vi "Do Turn.vi"(6 "Team in":refnum<class "Team.lvclass">, 7 "Round Number":u32, 9 "Neighbors":i32[](array[numeric]), 10 "Position":T1, 11 "Square in":refnum<class "Square.lvclass">) -> (2 "Run Result":T2, 3 "Square out":refnum<class "Square.lvclass">, 4 "Team out":refnum<class "Team.lvclass">)   [LabVIEW 2020, in "SquareBattle.lvlib" / "Square.lvclass"]
uses:
  Square.lvclass
  Run Result.ctl
  Action.ctl
  Direction.ctl
  Position.ctl
  Team/Team.lvclass
  Square.lvclass/Square.ctl
  SquareBattle.lvlib
panel:
  # "NW\nN\nNE\nE\nSE\nS\nSW\nW"
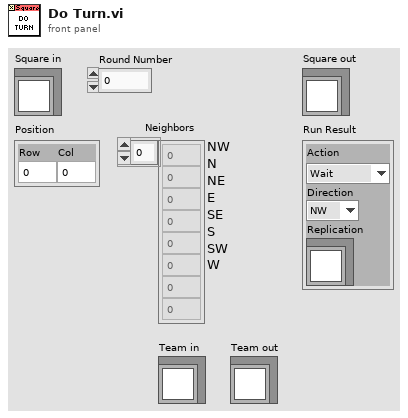
[diagram p1: front panel]
types:
  T1 = typedef "SquareBattle.lvlib/Position.ctl" = cluster{"Row":i32, "Col":i32}
  T2 = typedef "SquareBattle.lvlib/Run Result.ctl" = cluster{"Action":T3, "Direction":T4, "Replication":refnum<class "Square.lvclass">}
  T3 = typedef "SquareBattle.lvlib/Action.ctl" = enum16{"Wait", "Move", "Attack", "Replicate"}
  T4 = typedef "SquareBattle.lvlib/Direction.ctl" = enum16{"NW", "N", "NE", "E", "SE", "S", "SW", "W"}
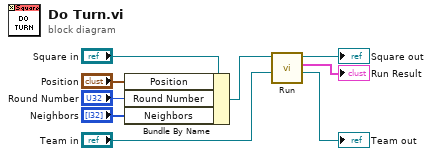
[diagram p0: block diagram]
diagram:
  n1 = Bundle By Name(cluster="Square in", "Position"="Position", "Round Number"="Round Number", "Neighbors"="Neighbors") -> (w4:refnum<class "Square.lvclass">)
  n2 = call-dynamic "Run.vi"("Team in"="Team in", "Square in"=w4) -> ("Team out"=→"Team out":refnum<class "Team.lvclass">, "Run Result"=→"Run Result":T2, "Square out"=→"Square out":refnum<class "Square.lvclass">)  [unwired: 7 in]
